vi "Check Overflow.vi"(8 "Bit":u8, 9 "Current Value":u32 format="%.0x", 10 "Previous Value":u32 format="%.0x", 11 "Backward?":bool) -> (2 "Crossed Halfway?":bool, 3 "Wrapped?":bool)   [LabVIEW 2015]
doc: "Compares the specified bit of the previous and current values to determine if it is different. If the bit changes from 0 to 1 when counting forward or from 1 to 0 when counting backward the <b>Crossed Halfway?</b> Boolean is TRUE. If the bit changes from 1 to 0 when counting up of from 0 to 1 when counting down the <b>Wrapped</b> Boolean is TRUE."
panel:
  # "Compares the specified bit of the previous and current values to determine if it is different. If the bit changes from 0 to 1 when counting forward or from 1 to 0 when counting backward the Crossed Halfway? Boolean is TRUE. If the bit changes from 1 to 0 when counting up of from 0 to 1 when counting down the Wrapped Boolean is TRUE."
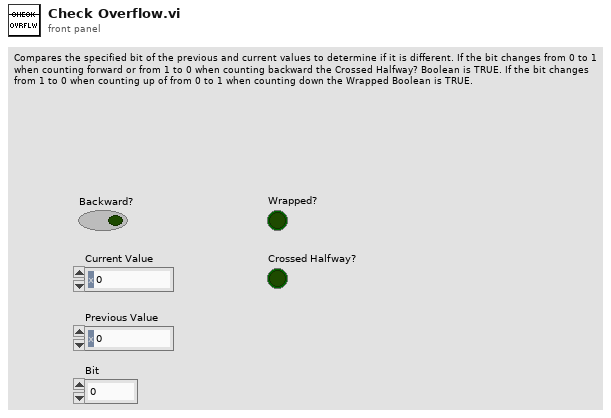
[diagram p1: front panel]
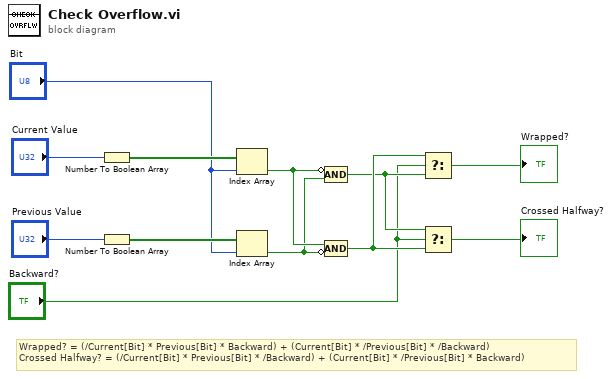
[diagram p0: block diagram]
diagram:
  # "Wrapped? = (/Current[Bit] * Previous[Bit] * Backward) + (Current[Bit] * /Previous[Bit] * /Backward)\nCrossed Halfway? = (/Current[Bit] * Previous[Bit] * /Backward) + (Current[Bit] * /Previous[Bit] * Backward)"
  n1 = Number To Boolean Array(number="Current Value") -> (Boolean array=w11:bool[])
  n2 = Number To Boolean Array(number="Previous Value") -> (Boolean array=w12:bool[])
  n3 = Index Array(array=w11, index="Bit") -> (element=w5:bool)
  n4 = Index Array(array=w12, index="Bit") -> (element=w4:bool)
  n5 = Compound Arithmetic op=AND(invert w5, w4) -> (w7:bool)
  n6 = Compound Arithmetic op=AND(w5, invert w4) -> (w8:bool)
  n7 = Select(t=w8, s="Backward?", f=w7) -> (s? t:f=→"Wrapped?":bool)
  n8 = Select(t=w7, s="Backward?", f=w8) -> (s? t:f=→"Crossed Halfway?":bool)
